vi "Exit.vi"(8 "error in (no error)":errorcluster, 11 "LNAX301 in":refnum<class "LNAX301.lvclass">) -> (0 "error out":errorcluster, 3 "LNAX301 out":refnum<class "LNAX301.lvclass">)   [LabVIEW 2017, in "LNAX301.lvclass"]
uses:
  LNAX301.lvclass
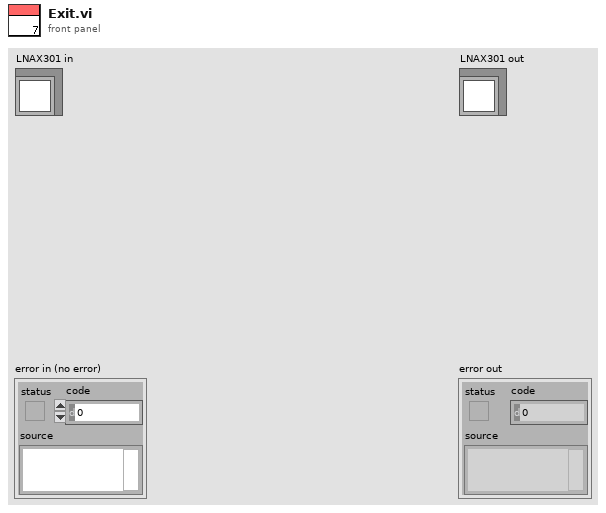
[diagram p1: front panel]
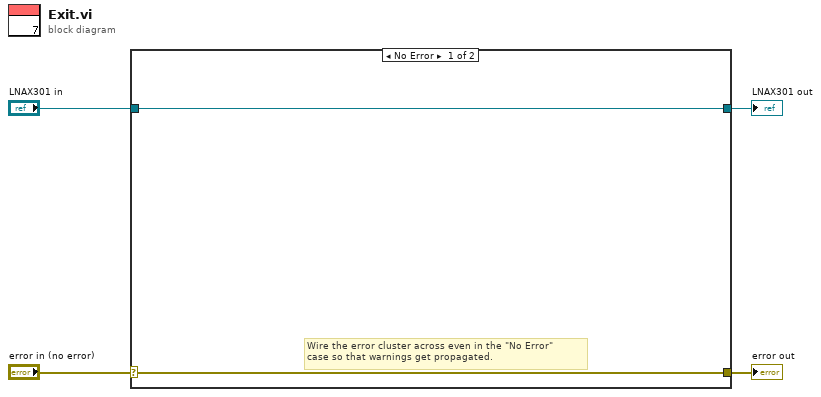
[diagram p0: block diagram]
diagram:
  n1 = case shown="No Error" "error in (no error)" {
    selector: "error in (no error)" -> [w5 w8]
    tunnel: [w5 w8] -> w3
    tunnel: [w6 w7] -> w1
    tunnel: "LNAX301 in" -> [w6 w7]
    frame No Error {
      # "Wire the error cluster across even in the \"No Error\"\ncase so that warnings get propagated."
    }
    frame Error {
    }
  }
  "error out" <- w3
  "LNAX301 out" <- w1
